vi "queue state & data (Array).vi"(6 "Priority Message Array? (F)":bool[](array[boolean]), 8 "error in (no error)":errorcluster, 9 "State Data Array":variant[](array[variant]), 10 "State Array":string[](array[string]), 11 "queue in":refnum<queue>) -> (0 "error out":errorcluster, 3 "queue out":refnum<queue>)   [LabVIEW 2015, in "queue state & data.lvlib"]
uses:
  queue state & data.lvlib
  controls/Message Cluster.ctl
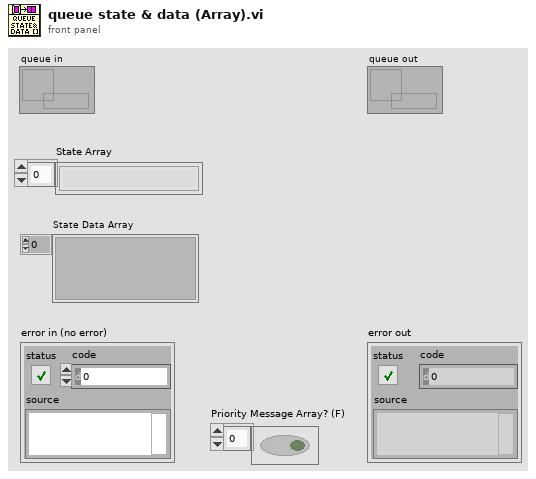
[diagram p1: front panel]
types:
  T1 = typedef "Message Cluster.ctl" = cluster{"Message":string, "Message Data":variant}
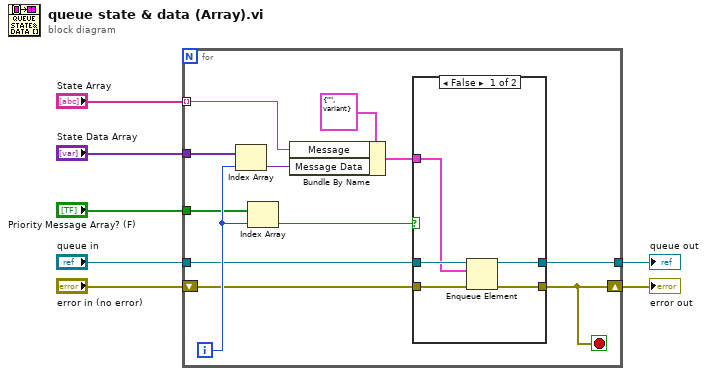
[diagram p0: block diagram]
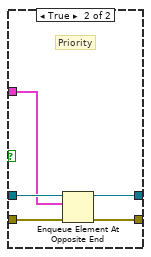
[diagram p2: hidden frame]
diagram:
  n1 = for {
    shift-right: [w15] -> w7
    shift-left: "error in (no error)" -> [w18]
    tunnel: "queue in" -> [w17]
    tunnel: [w16] -> w1
    tunnel: "Priority Message Array? (F)" -> [w14]
    tunnel: "State Data Array" -> [w12]
    tunnel: "State Array" -> [w11] mode=indexing
    i -> [w19]
    stop <- w15 stop-if-true
    n2 = Index Array(array=w12, index=w19) -> (element=w10:variant)
    n3 = Index Array(array=w14, index=w19) -> (element=w13:bool)
    n4 = Bundle By Name(cluster=T1 {"Message"="", "Message Data"=variant}, "Message"=w11, "Message Data"=w10) -> (w8:T1)
    n5 = case shown="False" w13 {
      tunnel: w18 -> [w24 w29]
      tunnel: w17 -> [w21 w27]
      tunnel: [w23 w26] -> w16
      tunnel: w8 -> [w20 w25]
      tunnel: [w22 w28] -> w15
      frame False {
        n6 = Enqueue Element(queue=w21, element=w20, error in (no error)=w24) -> (queue out=w23:refnum<queue>, error out=w22:errorcluster)  [unwired: 1 in, 1 out]
      }
      frame True {
        # "Priority"
        n7 = Enqueue Element At Opposite End(queue=w27, element=w25, error in (no error)=w29) -> (queue out=w26:refnum<queue>, error out=w28:errorcluster)  [unwired: 1 in, 1 out]
      }
    }
  }
  "error out" <- w7
  "queue out" <- w1
